vi "Initialize.vi"(6 "Pulse duration (ms)":u32=50, 8 "error in (no error)":errorcluster, 10 "TTL Ports":tag, 11 "TTL in":refnum<class "TTL.lvclass">) -> (0 "error out":errorcluster, 3 "TTL out":refnum<class "TTL.lvclass">)   [LabVIEW 2014, in "TTL.lvclass"]
uses:
  TTL.lvclass
  Program Files/National Instruments/LabVIEW 2011/resource/objmgr/daqmx.rc
  <vilib>/DAQmx/create/channels.llb/DAQmx Create Channel (DO-Digital Output).vi
  TTL Status Data.ctl
panel:
  in  "TTL Status Data":T1
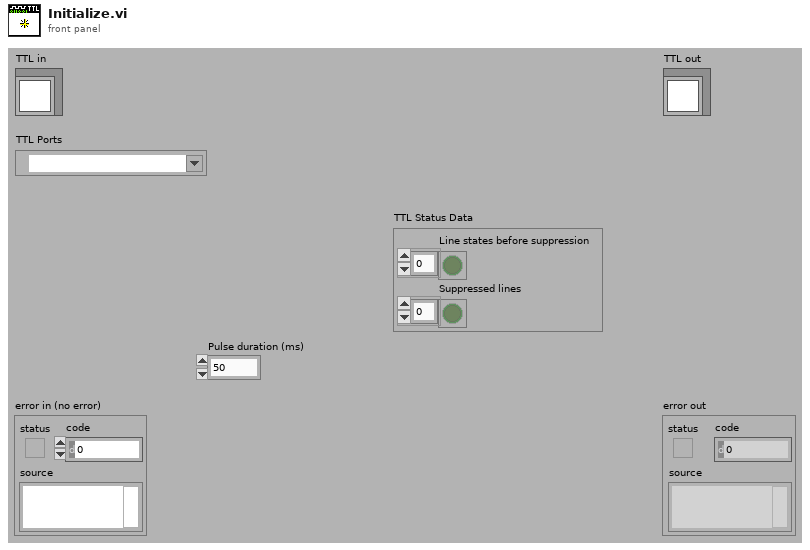
[diagram p1: front panel]
types:
  T1 = typedef "TTL.lvclass/TTL Status Data.ctl" = cluster{"Line states before suppression":bool[], "Suppressed lines":bool[]}
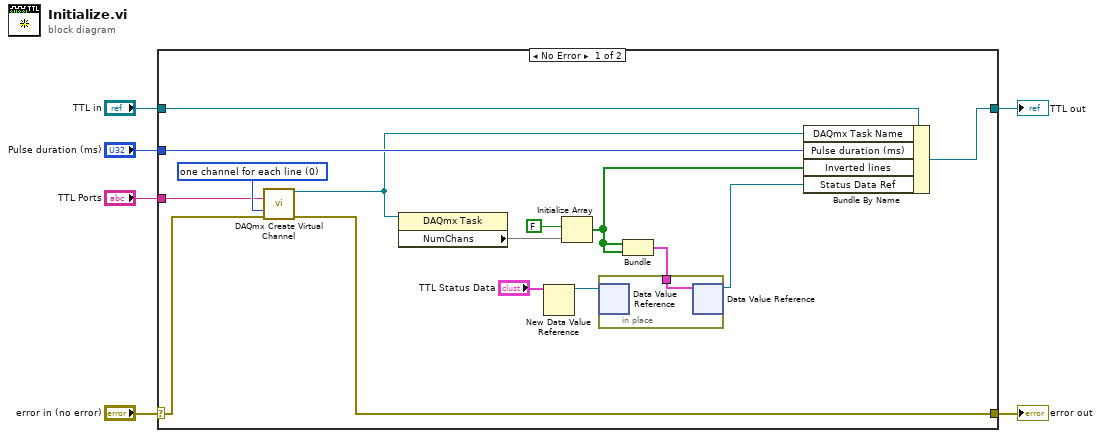
[diagram p0: block diagram]
diagram:
  n1 = case shown="No Error" "error in (no error)" {
    selector: "error in (no error)" -> [w18 w24]
    tunnel: [w15 w24] -> w5
    tunnel: [w16 w23] -> w3
    tunnel: "TTL in" -> [w19 w23]
    tunnel: "TTL Ports" -> [w20 _]
    tunnel: "Pulse duration (ms)" -> [w17 _]
    frame No Error {
      w21 = 0 items=["one channel for each line", "one channel for all lines"] ("line grouping")
      n2 = call-poly <vilib>:"DAQmx Create Virtual Channel.vi"("lines"=w20, "line grouping"=w21, "error in"=w18) -> ("task out"=w13:refnum<k21>, "error out"=w15:errorcluster)  [unwired: 11 in]
      n3 = property class="DAQmx Task"(reference=w13) -> ("NumChans"=w12)  [unwired: 1 in, 2 out]
      n4 = New Data Value Reference(data value="TTL Status Data") -> (data value reference=w9:refnum<data-value>)  [unwired: 1 in, 1 out]
      n5 = Initialize Array(FALSE, w12) -> (w11:bool[])
      n6 = Bundle(w11, w11) -> (w8:cluster{bool[], bool[]})  [unwired: 1 in]
      n7 = in-place {
        in-place-border: w8 -> [w22]
        n8 = in-place-dvr #1(w9) -> ()  [unwired: 2 out]
        n9 = in-place-dvr #1(w22) -> (w7:refnum<data-value>)  [unwired: 1 out]
      }
      n10 = Bundle By Name(cluster=w19, "DAQmx Task Name"=w13, "Pulse duration (ms)"=w17, "Inverted lines"=w11, "Status Data Ref"=w7) -> (w16:refnum<class "TTL.lvclass">)
    }
    frame Error {
    }
  }
  "error out" <- w5
  "TTL out" <- w3
